vi "KE26XX Factory Pulse Usage.vi"(0 "VISA resource name":refnum<visa-resource-name>, 1 "Read Byte Count":u32=1024, 2 "Timeout Value":u32=20000, 3 "Error Query (False)":bool, 4 "Channel (Channel A)":T1, 5 "error in (no error)":errorcluster, 6 "Bias (Volts)":dbl, 7 "On Time (s)":dbl=0.005, 8 "Level (Volts)":dbl=5.0, 9 "Off Time (s)":dbl=0.005, 10 "Limit (Amps)":dbl=0.01, 11 "Pulse Points":u32=10, 12 "Sense (2 Wire)":enum32{"2 Wire", "4 Wire", "Calibration"}(ring), 13 "Tag":u32=1 min=1) -> (15 "Success":bool, 16 "Message":string, 18 "Buffer Data":string, 19 "error out":errorcluster)   [LabVIEW 2012]
doc: "This example shows how to use the Factory Pulse Functions.\n\nThis example demonstrates the following:\n• How to configure a voltage pulse\n• How to run a single channel pulse test\n• How to create volatile reading buffers\n• How to configure reading buffers\n• How to place reading buffers in a table for dual measurements during pulsing\n• How to configure the SourceMeter for pulse operation.\n\n<b>Remarks::</b>\nIf you get a query interrupted error after running this VI, but the pulse test appears to be successful and data has been returned, then you probably have your <b>Read Byte Count</b> set too low to get all the data back."
uses:
  Keithley 2600 Series.lvlib
  Public/Channel.ctl
panel:
  in  "Measure Range":dbl=0.01
  in  "NPLC":dbl=0.001
  # "(c) 2008 Keithley Instruments, Inc.  ALL RIGHTS RESERVED."
  # "Pulse Parameters"
  # "Measurement Settings"
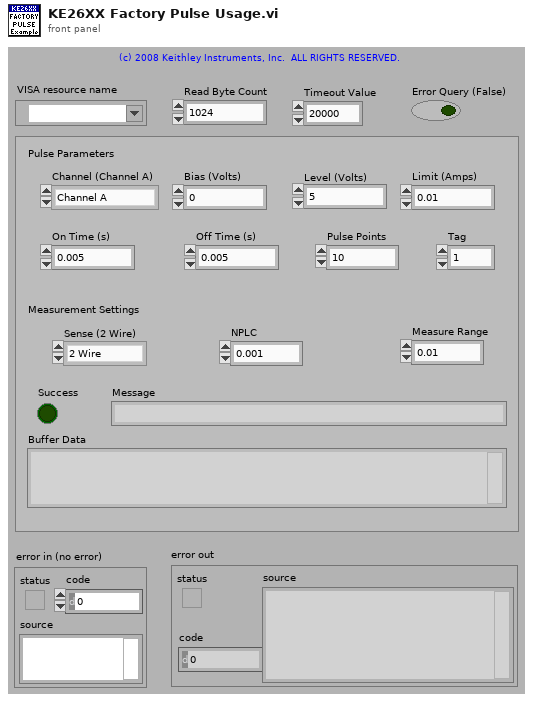
[diagram p1: front panel]
types:
  T1 = typedef "Keithley 2600 Series.lvlib/Channel.ctl" = enum32{"Channel A", "Channel B"}
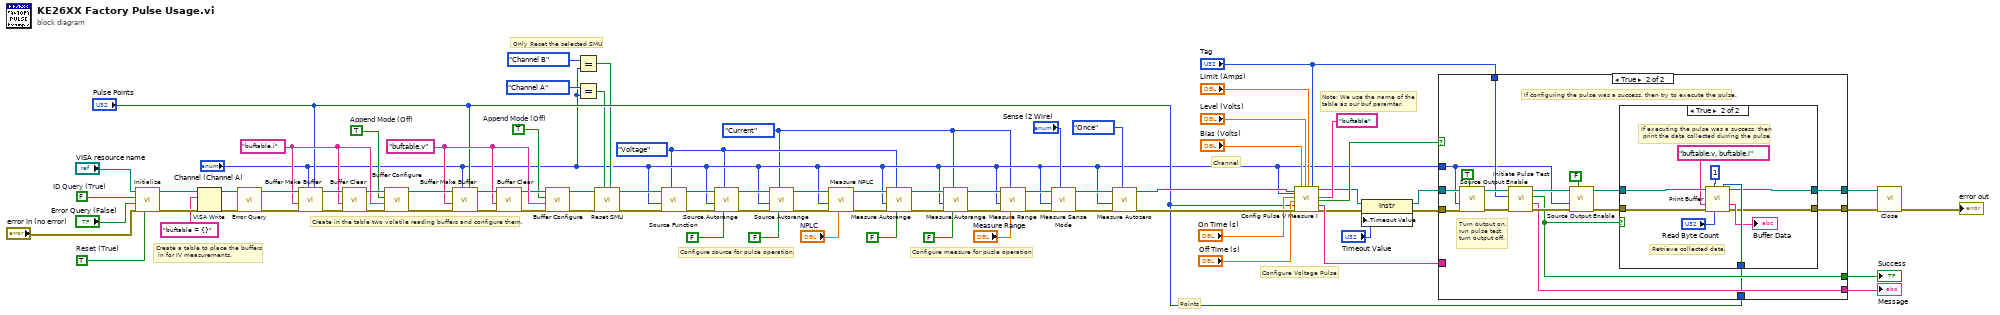
[diagram p0: block diagram]
diagram:
  w1 = enum32{"Current", "Voltage"}."Current" ("Function (Current)")
  w2 = enum32{"Current", "Voltage"}."Voltage" ("Function (Current)")
  w25 = FALSE  # ID Query (True)
  w29 = TRUE  # Reset (True)
  w55 = TRUE  # Append Mode (Off)
  w58 = "buftable.v" ("Buffer Name (buf)")
  w64 = TRUE  # Append Mode (Off)
  w63 = "buftable.i" ("Buffer Name (buf)")
  # "Only Reset the selected SMU"
  # "Note: We use the name of the\ntable as our buf paramter."
  # "Configure Voltage Pulse"
  # "Configure measure for pusle operation"
  # "Configure source for pulse operation"
  # "Create in the table two volatile reading buffers and configure them."
  # "Create a table to place the buffers\n in for IV measurements."
  # "Points"
  # "Channel"
  n1 = call "Initialize.vi"("Reset (True)"=w29, "error in (no error)"="error in (no error)", "Error Query (False)"="Error Query (False)", "ID Query (True)"=w25, "VISA resource name"="VISA resource name") -> ("error out"=w74:errorcluster, "VISA resource name out"=w75:refnum<visa-resource-name>)  [unwired: 1 in, 4 out]
  n2 = VISA Write(VISA resource name=w75, write buffer="buftable = {}", error in (no error)=w74) -> (VISA resource name out=w72:refnum<visa-resource-name>, error out=w71:errorcluster)  [unwired: 1 out]
  n3 = call "Error Query.vi"("error in (no error)"=w71, "VISA resource name"=w72) -> ("error out"=w69:errorcluster, "VISA resource name out"=w70:refnum<visa-resource-name>)  [unwired: 8 out]
  n4 = call "Buffer Make Buffer.vi"("Capacity (1)"="Pulse Points", "Channel (Channel A)"="Channel (Channel A)", "error in (no error)"=w69, "Buffer Name (buf)"=w63, "VISA resource name"=w70) -> ("error out"=w68:errorcluster, "VISA resource name out"=w67:refnum<visa-resource-name>)  [unwired: 1 in, 4 out]
  n5 = call "Buffer Clear.vi"("error in (no error)"=w68, "Buffer Name"=w63, "VISA resource name"=w67) -> ("error out"=w65:errorcluster, "VISA resource name out"=w66:refnum<visa-resource-name>)  [unwired: 7 out]
  n6 = call "Buffer Configure.vi"("error in (no error)"=w65, "Buffer Name"=w63, "Append Mode (Off)"=w64, "VISA resource name"=w66) -> ("error out"=w61:errorcluster, "VISA resource name out"=w62:refnum<visa-resource-name>)  [unwired: 3 in, 3 out]
  n7 = call "Buffer Make Buffer.vi"("Capacity (1)"="Pulse Points", "Channel (Channel A)"="Channel (Channel A)", "error in (no error)"=w61, "Buffer Name (buf)"=w58, "VISA resource name"=w62) -> ("error out"=w59:errorcluster, "VISA resource name out"=w60:refnum<visa-resource-name>)  [unwired: 1 in, 4 out]
  n8 = call "Buffer Clear.vi"("error in (no error)"=w59, "Buffer Name"=w58, "VISA resource name"=w60) -> ("error out"=w56:errorcluster, "VISA resource name out"=w57:refnum<visa-resource-name>)  [unwired: 7 out]
  n9 = call "Buffer Configure.vi"("error in (no error)"=w56, "Buffer Name"=w58, "Append Mode (Off)"=w55, "VISA resource name"=w57) -> ("error out"=w54:errorcluster, "VISA resource name out"=w53:refnum<visa-resource-name>)  [unwired: 3 in, 3 out]
  n10 = Equal?(x=enum32{"Channel A", "Channel B"}."Channel B", y="Channel (Channel A)") -> (x = y?=w4:bool)
  n11 = Equal?(x=enum32{"Channel A", "Channel B"}."Channel A", y="Channel (Channel A)") -> (x = y?=w5:bool)
  n12 = call "Reset SMU.vi"("SMU B (No)"=w4, "SMU A (No)"=w5, "error in (no error)"=w54, "VISA resource name"=w53) -> ("error out"=w52:errorcluster, "VISA resource name out"=w81:refnum<visa-resource-name>)  [unwired: 1 in, 5 out]
  n13 = call "Source Function.vi"("Function (Current)"=w2, "error in (no error)"=w52, "Channel (Channel A)"="Channel (Channel A)", "VISA resource name"=w81) -> ("error out"=w51:errorcluster, "VISA resource name out"=w80:refnum<visa-resource-name>)  [unwired: 2 in, 4 out]
  n14 = call "Source Autorange.vi"("Autorange (On)"=FALSE, "Function (Current)"=w2, "error in (no error)"=w51, "Channel (Channel A)"="Channel (Channel A)", "VISA resource name"=w80) -> ("error out"=w22:errorcluster, "VISA resource name out"=w23:refnum<visa-resource-name>)  [unwired: 1 in, 4 out]
  n15 = call "Source Autorange.vi"("Autorange (On)"=FALSE, "Function (Current)"=w1, "error in (no error)"=w22, "Channel (Channel A)"="Channel (Channel A)", "VISA resource name"=w23) -> ("error out"=w8:errorcluster, "VISA resource name out"=w9:refnum<visa-resource-name>)  [unwired: 1 in, 4 out]
  n16 = call "Measure NPLC.vi"("NPLC (1.000)"="NPLC", "error in (no error)"=w8, "Channel (Channel A)"="Channel (Channel A)", "VISA resource name"=w9) -> ("error out"=w50:errorcluster, "VISA resource name out"=w79:refnum<visa-resource-name>)  [unwired: 1 in, 5 out]
  n17 = call "Measure Autorange.vi"("Autorange (On)"=FALSE, "Function (Current)"=w2, "error in (no error)"=w50, "Channel (Channel A)"="Channel (Channel A)", "VISA resource name"=w79) -> ("error out"=w17:errorcluster, "VISA resource name out"=w16:refnum<visa-resource-name>)  [unwired: 1 in, 4 out]
  n18 = call "Measure Autorange.vi"("Autorange (On)"=FALSE, "Function (Current)"=w1, "error in (no error)"=w17, "Channel (Channel A)"="Channel (Channel A)", "VISA resource name"=w16) -> ("error out"=w18:errorcluster, "VISA resource name out"=w19:refnum<visa-resource-name>)  [unwired: 1 in, 4 out]
  n19 = call "Measure Range.vi"("Range (1.000)"="Measure Range", "Function (Current)"=w1, "error in (no error)"=w18, "Channel (Channel A)"="Channel (Channel A)", "VISA resource name"=w19) -> ("error out"=w49:errorcluster, "VISA resource name out"=w78:refnum<visa-resource-name>)  [unwired: 1 in, 4 out]
  n20 = call "Measure Sense Mode.vi"("Sense (2 Wire)"="Sense (2 Wire)", "error in (no error)"=w49, "Channel (Channel A)"="Channel (Channel A)", "VISA resource name"=w78) -> ("error out"=w48:errorcluster, "VISA resource name out"=w77:refnum<visa-resource-name>)  [unwired: 1 in, 5 out]
  n21 = call "Measure Autozero.vi"("Autozero (Auto)"=enum32{"Off", "Once", "Auto"}."Once", "error in (no error)"=w48, "Channel (Channel A)"="Channel (Channel A)", "VISA resource name"=w77) -> ("error out"=w47:errorcluster, "VISA resource name out"=w76:refnum<visa-resource-name>)  [unwired: 1 in, 5 out]
  n22 = call "Config Pulse V Measure I.vi"("VISA resource name"=w76, "Channel (Channel A)"="Channel (Channel A)", "On Time"="On Time (s)", "Off Time"="Off Time (s)", "Points (1)"="Pulse Points", "error in"=w47, "Bias (0)"="Bias (Volts)", "Level"="Level (Volts)", "Limit"="Limit (Amps)", "Tag (1)"="Tag", "Buffer (nil)"="buftable") -> ("VISA resource name out"=w14:refnum<visa-resource-name>, "Success"=w37:bool, "Message"=w34:string, "error out"=w12:errorcluster)  [unwired: 1 in, 4 out]
  n23 = property class="Instr"(reference=w14, error in=w12, "General Settings:Timeout Value"="Timeout Value") -> (reference out=w13:refnum<visa-resource-name>, error out=w11:errorcluster)
  n24 = case shown="True" w37 {
    selector: w37 -> [w87 _]
    tunnel: w13 -> [w85 w104]
    tunnel: w11 -> [w84 w101]
    tunnel: "Tag" -> [_ w98]
    tunnel: "Channel (Channel A)" -> [_ w95]
    tunnel: [w85 w92] -> w36
    tunnel: [w84 w91] -> w35
    tunnel: w34 -> [w86 _]
    tunnel: [w87 w90] -> w33
    tunnel: [w86 w89] -> w32
    tunnel: "Pulse Points" -> [_ w88]
    frame False {
      # "If configuring the pulse failed, then there is no point in attempting to execute\nthe pulse so just output the failure message and close."
    }
    frame True {
      # "Turn output on,\nrun pulse test,\nturn output off."
      # "If configuring the pulse was a success, then try to execute the pulse."
      n25 = call "Source Output Enable.vi"("Output (Off)"=TRUE, "error in (no error)"=w101, "Channel (Channel A)"=w95, "VISA resource name"=w104) -> ("error out"=w100:errorcluster, "VISA resource name out"=w103:refnum<visa-resource-name>)  [unwired: 1 in, 5 out]
      n26 = call "Initiate Pulse Test.vi"("error in"=w100, "Tag"=w98, "VISA resource name"=w103) -> ("error out"=w99:errorcluster, "Message"=w89:string, "Success"=w90:bool, "VISA resource name out"=w102:refnum<visa-resource-name>)  [unwired: 1 in, 4 out]
      n27 = call "Source Output Enable.vi"("Output (Off)"=FALSE, "error in (no error)"=w99, "Channel (Channel A)"=w95, "VISA resource name"=w102) -> ("error out"=w93:errorcluster, "VISA resource name out"=w94:refnum<visa-resource-name>)  [unwired: 1 in, 5 out]
      n28 = case shown="True" w90 {
        tunnel: w94 -> [w105 w115]
        tunnel: w93 -> [w106 w114]
        tunnel: [w105 w109] -> w92
        tunnel: [w106 w108] -> w91
        tunnel: w88 -> [_ w112]
        frame False {
          # "If executing the pulse failed, then don't try to\nprint back the data as the buffers will be empty."
        }
        frame True {
          # "Retrieve collected data."
          # "If executing the pulse was a success, then\n print the data collected durring the pulse."
          n29 = call "Print Buffer.vi"("VISA resource name"=w115, "Start Index (1)"=u32 1, "End Index (1)"=w112, "Buffer Name(s)"="buftable.v, buftable.i" ("Buffer Name(s) (smua.nvbuffer1)"), "error in (no error)"=w114, "Byte Count (1024)"="Read Byte Count") -> ("VISA resource name out"=w109:refnum<visa-resource-name>, "Buffer Data"=→"Buffer Data":string, "error out"=w108:errorcluster)  [unwired: 1 in, 6 out]
        }
      }
    }
  }
  "Message" <- w32
  "Success" <- w33
  n30 = call "Close.vi"("error in (no error)"=w35, "VISA resource name"=w36) -> ("error out"=→"error out":errorcluster)  [unwired: 9 out]
